vi "detectedFreq.vi"(0 "Interface in":T1, 9 "timeout (5000 ms)":i32=5000, 11 "error in":errorcluster) -> (4 "Interface out":T1, 6 "detectedFreq":sgl, 15 "error out":errorcluster)   [LabVIEW 2017, in "ThreePhasePLLInterface.lvlib"]
uses:
  ThreePhasePLLInterface.lvlib
  InterfaceRef.ctl
  <instrlib>/_niInstr/Instruction Framework/v1/Host/Instruction Target/niInstr Instruction Target v1 Host.lvclass
  <instrlib>/_niInstr/Instruction Framework/v1/Host/Instruction Framework Context/niInstr Instruction Framework Context v1 Host.lvclass
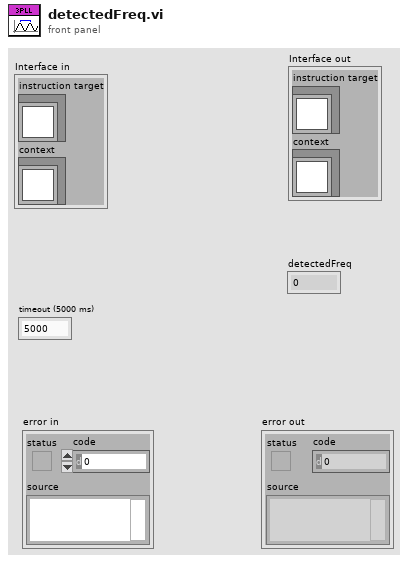
[diagram p1: front panel]
types:
  T1 = typedef "ThreePhasePLLInterface.lvlib/InterfaceRef.ctl" = cluster{"instruction target":refnum<class "niInstr Instruction Target v1 Host.lvclass">, "context":refnum<class "niInstr Instruction Framework Context v1 Host.lvclass">}
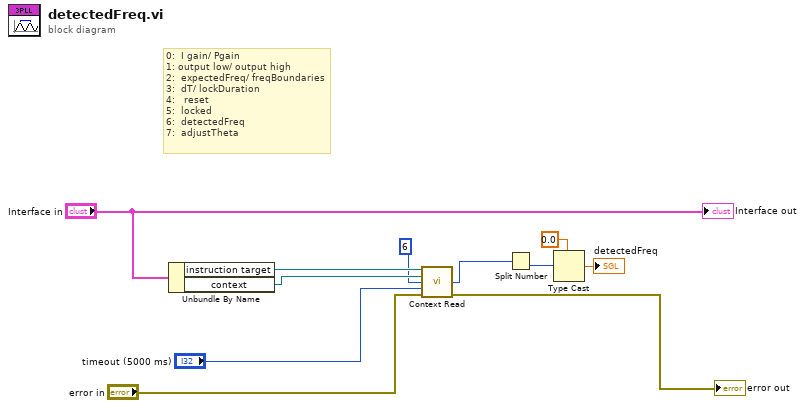
[diagram p0: block diagram]
diagram:
  # "0:  I gain/ Pgain\n1: output low/ output high\n2:  expectedFreq/ freqBoundaries\n3:  dT/ lockDuration\n4:   reset\n5:  locked\n6:  detectedFreq\n7:  adjustTheta"
  n1 = Unbundle By Name("Interface in") -> ("instruction target"=w11:refnum<class "niInstr Instruction Target v1 Host.lvclass">, "context"=w10:refnum<class "niInstr Instruction Framework Context v1 Host.lvclass">)
  n2 = call <instrlib>:"Context Read.vi"("instruction target in"=w11, "context in"=w10, "address"=u64 6, "timeout (5000 ms)"="timeout (5000 ms)", "error in"="error in") -> ("data"=w4:u64, "error out"=→"error out":errorcluster)  [unwired: 7 in, 2 out]
  n3 = Split Number(x=w4) -> (lo(x)=w3:u32)  [unwired: 1 out]
  n4 = Type Cast(type=sgl 0.0, x=w3) -> (*(type *) &x=→"detectedFreq":sgl)
  "Interface out" <- "Interface in"
